vi "makeNames.vi"(11 "Strings":string[](array[string])) -> (3 "Names":string[](array[string]))   [LabVIEW 2012]
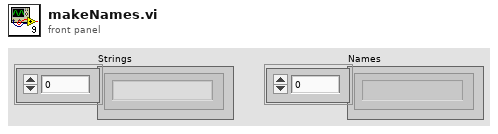
[diagram p1: front panel]
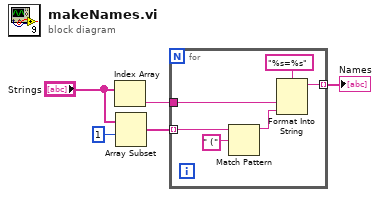
[diagram p0: block diagram]
diagram:
  n1 = Index Array(array="Strings") -> (element=w1:string)  [unwired: 1 in]
  n2 = Array Subset(array="Strings", index=1) -> (w2:string[])  [unwired: 1 in]
  n3 = for {
    tunnel: w2 -> [w10] mode=indexing
    tunnel: [w7] -> w4 mode=indexing
    tunnel: w1 -> [w9]
    n4 = Match Pattern(string=w10, regular expression=" (") -> (before substring=w6:string)  [unwired: 4 out]
    n5 = Format Into String(format string="%s=%s", w9, w6) -> (resulting string=w7:string)  [unwired: 2 in, 1 out]
  }
  "Names" <- w4
